vi "Order of Polynomial (DBL).vi"(11 "P(x)":dbl[](array[numeric]) min=0.0 max=127.0 format="%#.6g") -> (0 "error":i32, 3 "order":i32)   [LabVIEW 2020, in "NI_AALPro.lvlib"]
doc: "Finds the order, or polynomial degree, of polynomial <B>P(x)</B>. Wire data to the <B>P(x)</B> input to determine the polymorphic instance to use or manually select the instance."
uses:
  NI_AALPro.lvlib
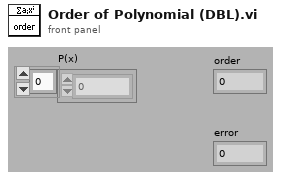
[diagram p1: front panel]
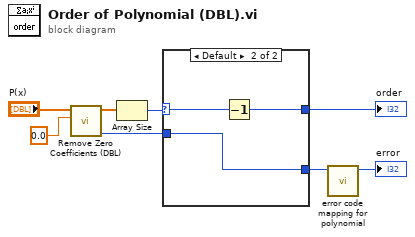
[diagram p0: block diagram]
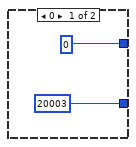
[diagram p2: hidden frame]
diagram:
  n1 = call "Remove Zero Coefficients (DBL).vi"("threshold"=0.0, "P(x) In"="P(x)") -> ("error"=w3:i32, "P(x) Out"=w5:dbl[])  [unwired: 7 in, 1 out]
  n2 = Array Size(array=w5) -> (size(s)=w7:i32)
  n3 = case shown="Default" w7 {
    selector: w7 -> [_ w13]
    tunnel: [0 w12] -> w8
    tunnel: [20003 ("empty array") w11] -> w2
    tunnel: w3 -> [_ w11]
    frame 0 {
    }
    frame Default {
      n4 = Decrement(x=w13) -> (x-1=w12:i32)
    }
  }
  "order" <- w8
  n5 = call "error code mapping for polynomial.vi"("error in"=w2) -> ("error out"=→"error":i32)  [unwired: 10 in]
